vi "Chamber Status Updated.vi"(6 "Heater State":T1, 8 "error in (no error)":errorcluster, 9 "Temperature Ramp Rate":dbl, 10 "Temperature Set Point":dbl, 11 "Actual Temperature":dbl) -> (0 "error out":errorcluster)   [LabVIEW 2015, in "Thermal Chamber Controller_DQMH.lvlib"]
doc: "Request the Thermal Chamber Controller to Update the Chamber Status. \nBroadcast to any VI registered to listen to Thermal Chamber Controller's broadcast events that the Chamber Status was updated.\n_____\nCreated using Delacor QMH Event Scripter 1.0.0.50.\n____\nDelacor QMH Thermal Chamber Examples 4.0.0.21\nCopyright (c) 2018, Delacor"
uses:
  Thermal Chamber Controller_DQMH.lvlib
  Heater State--enum.ctl
  Update Chamber Status Argument--cluster.ctl
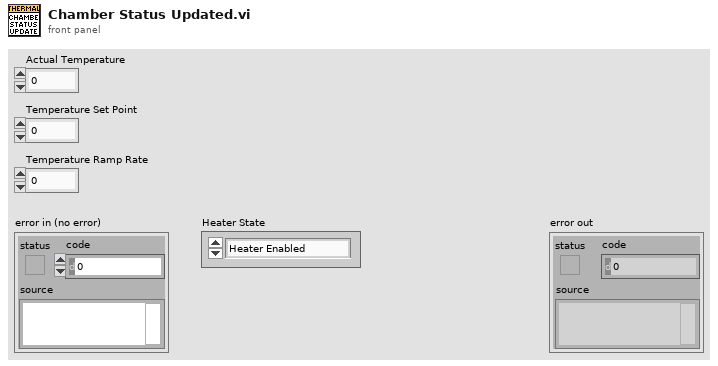
[diagram p1: front panel]
types:
  T1 = typedef "Thermal Chamber Controller_DQMH.lvlib/Heater State--enum.ctl" = enum16{"Heater Enabled", "Heater Disabled"}
  T2 = typedef "Thermal Chamber Controller_DQMH.lvlib/Update Chamber Status Argument--cluster.ctl" = cluster{"Temperature Set Point":dbl, "Temperature Ramp Rate":dbl, "Heater State":T1, "Actual Temperature":dbl}
  T3 = typedef "Thermal Chamber Controller_DQMH.lvlib/Broadcast Events--cluster.ctl" = cluster{"Module Did Init":refnum<user-event>, "Status Updated":refnum<user-event>, "Error Reported":refnum<user-event>, "Module Did Stop":refnum<user-event>, "Update Module Execution Status":refnum<user-event>, "Set Point Updated":refnum<user-event>, "Ramp Rate Updated":refnum<user-event>, "Heater State Updated":refnum<user-event>, "Chamber Status Updated":refnum<user-event>}
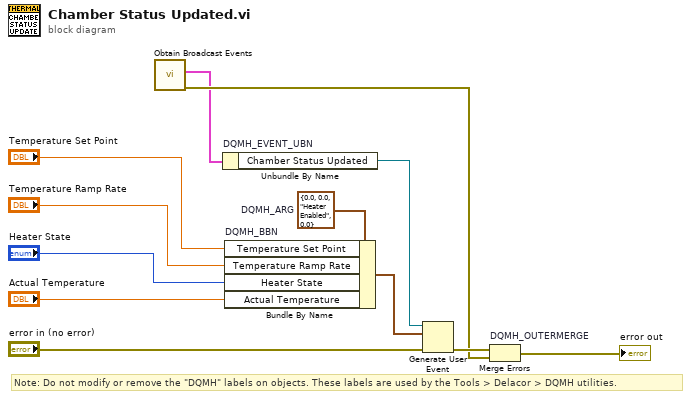
[diagram p0: block diagram]
diagram:
  w7 = T2 {"Temperature Set Point"=0.0, "Temperature Ramp Rate"=0.0, "Heater State"=enum."Heater Enabled", "Actual Temperature"=0.0}  # DQMH_ARG
  # "Note: Do not modify or remove the \"DQMH\" labels on objects. These labels are used by the Tools > Delacor > DQMH utilities."
  n1 = call "Obtain Broadcast Events.vi"() -> ("error out"=w2:errorcluster, "Thermal Chamber Controller_DQMH Broadcast Events"=w1:T3)  [unwired: 10 in]
  n2 = Unbundle By Name "DQMH_EVENT_UBN"(w1) -> ("Chamber Status Updated"=w8:refnum<user-event>)
  n3 = Bundle By Name "DQMH_BBN"(cluster=w7, "Temperature Set Point"="Temperature Set Point", "Temperature Ramp Rate"="Temperature Ramp Rate", "Heater State"="Heater State", "Actual Temperature"="Actual Temperature") -> (w9:T2)
  n4 = Generate User Event(user event=w8, event data cluster=w9, error in="error in (no error)") -> (error out=w10:errorcluster)  [unwired: 1 in, 1 out]
  n5 = Merge Errors "DQMH_OUTERMERGE"(w10, w2) -> (→"error out":errorcluster)
